vi "Write Resources.vi"(9 "Resources":T1, 11 "Bank in":refnum<class "Bank.lvclass">) -> (3 "Bank out":refnum<class "Bank.lvclass">)   [LabVIEW 2019, in "Bank.lvclass"]
uses:
  Bank.lvclass
  DIO Resources.ctl
  Bank.lvclass/Bank.ctl
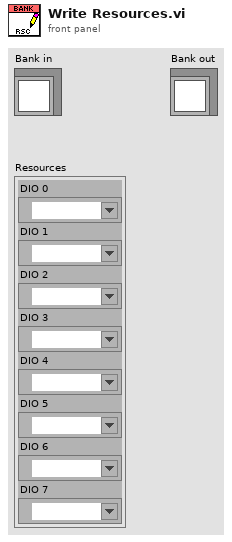
[diagram p1: front panel]
types:
  T1 = typedef "Bank.lvclass/DIO Resources.ctl" = cluster{"DIO 0":refnum<k21>, "DIO 1":refnum<k21>, "DIO 2":refnum<k21>, "DIO 3":refnum<k21>, "DIO 4":refnum<k21>, "DIO 5":refnum<k21>, "DIO 6":refnum<k21>, "DIO 7":refnum<k21>}
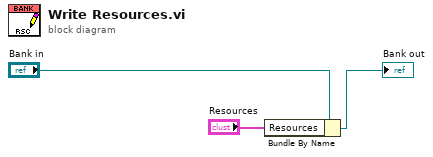
[diagram p0: block diagram]
diagram:
  n1 = Bundle By Name(cluster="Bank in", "Resources"="Resources") -> (→"Bank out":refnum<class "Bank.lvclass">)
